vi "Rectangular To Polar.vi"(2 "y":dbl format="%0.2f", 3 "x":dbl format="%0.2f") -> (0 "phase":dbl format="%0.2f", 1 "magnitude":dbl format="%0.2f")   [LabVIEW 2020, in "NI_AALPro.lvlib"]
doc: "Converts the rectangular coordinates represented by the input values, x and y, to polar coordinates."
uses:
  NI_AALPro.lvlib
panel:
  # "Rectangular To Polar"
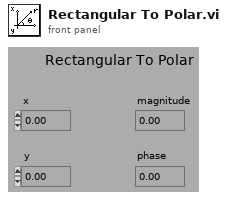
[diagram p1: front panel]
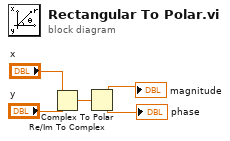
[diagram p0: block diagram]
diagram:
  n1 = Re/Im To Complex(1:"y", 2:"x") -> (0:w3:cdb)
  n2 = Complex To Polar(r * e^(i*theta)=w3) -> (r=→"magnitude":dbl, theta=→"phase":dbl)
